vi "Assert Error Code.vi"(6 "clear all error codes":bool, 8 "error in":errorcluster, 9 "additional info to prepend":string, 10 "expected error description":string, 11 "expected error code":i32) -> (0 "error out":errorcluster, 2 "details":string, 3 "error code match?":bool)   [LabVIEW 2020, in "MeasurementServerTests.lvlib"]
uses:
  MeasurementServerTests.lvlib
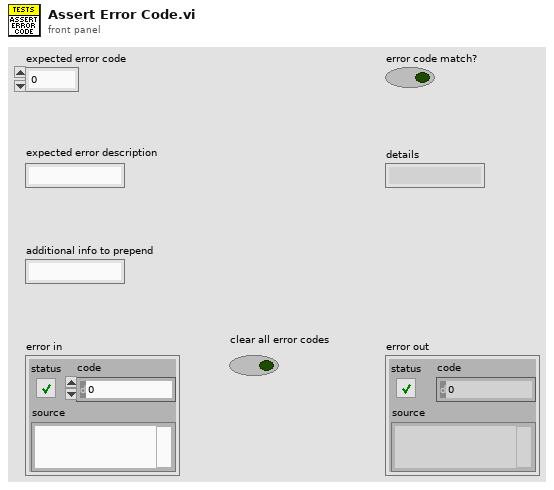
[diagram p1: front panel]
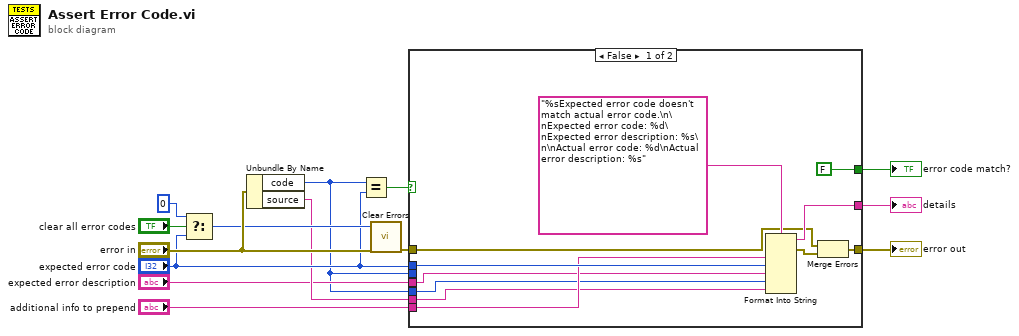
[diagram p0: block diagram]
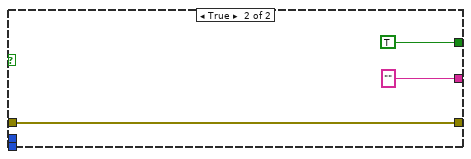
[diagram p2: hidden frame]
diagram:
  n1 = Select(t=0, s="clear all error codes", f="expected error code") -> (s? t:f=w6:i32)
  n2 = Unbundle By Name("error in") -> ("code"=w1:i32, "source"=w3:string)
  n3 = Equal?(x=w1, y="expected error code") -> (x = y?=w11:bool)
  n4 = call <vilib>:"Clear Errors.vi"("error in (no error)"="error in", "specific error code to clear (0: all)"=w6) -> ("error out"=w10:errorcluster)  [unwired: 4 in, 1 out]
  n5 = case shown="False" w11 {
    tunnel: [FALSE TRUE] -> w13
    tunnel: [w23 "" ("result")] -> w14
    tunnel: w10 -> [w18 w26]
    tunnel: [w20 w26] -> w9
    tunnel: "expected error code" -> [w22 _]
    tunnel: w1 -> [_ _]
    tunnel: "additional info to prepend" -> [w21 _]
    tunnel: w3 -> [w15 _]
    tunnel: "expected error description" -> [w17 _]
    tunnel: w1 -> [w16 _]
    frame False {
      n6 = Format Into String(format string="%sExpected error code doesn't match actual error code.\n\nExpected error code: %d\nExpected error description: %s\n\nActual error code: %d\nActual error description: %s" ("result"), w21, w22, w17, w16, w15) -> (resulting string=w23:string, error out=w19:errorcluster)  [unwired: 2 in]
      n7 = Merge Errors(w18, w19) -> (w20:errorcluster)
    }
    frame True {
    }
  }
  "error out" <- w9
  "details" <- w14
  "error code match?" <- w13
